vi "Write HDF5.vi"(4 "Append? [F]":bool, 6 "Igor Commands":string, 7 "path":path, 8 "error in (no error)":errorcluster, 9 "Comments":string, 10 "Data (Dictionary)":T1[](array[typedef]), 11 "LV to ITX.lvclass":refnum<class "LV to ITX.lvclass">) -> (0 "error out":errorcluster, 2 "path 2":path, 3 "LV to ITX.lvclass":refnum<class "LV to ITX.lvclass">)   [LabVIEW 2016, in "LV to ITX.lvclass"]
uses:
  LV to ITX.lvclass
  Typedefs/Dictionary--cluster.ctl
  <vilib>/addons/h5labview2/file/H5Fmode.ctl
  Typedefs/Filetype--enum.ctl
  LV to ITX.lvclass/LV to ITX.ctl
  <vilib>/addons/h5labview2/base/lib_path.vi
  <vilib>/addons/h5labview2/base/H5Equery.vi
  <vilib>/addons/h5labview2/base/hid_t.ctl
  <vilib>/addons/h5labview2/dataset/H5Dwrite.llb/H5Dwrite.xnode
  <vilib>/addons/h5labview2/file/H5F.lvlib
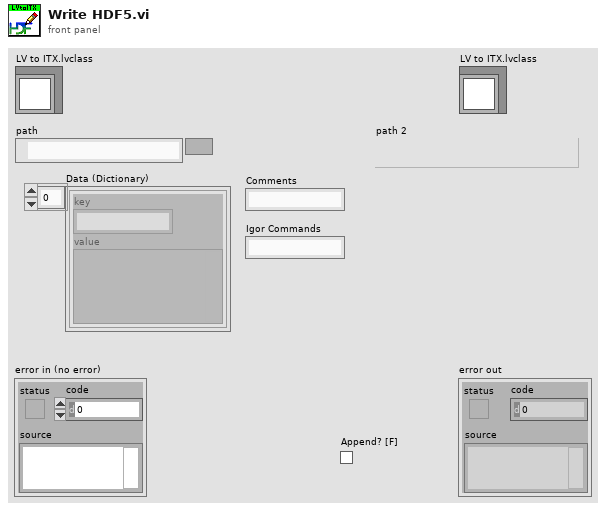
[diagram p1: front panel]
types:
  T1 = typedef "LV to ITX.lvclass/Dictionary--cluster.ctl" = cluster{"key":string, "value":variant}
  T2 = typedef "LV to ITX.lvclass/Filetype--enum.ctl" = enum16{"DAT", "ITX", "HDF5", "TDMS", "VI"}
  T3 = typedef "H5F.lvlib/H5Fmode.ctl" = enum16{"read-only", "read-write", "overwrite", "create new", "open or create"}
  T4 = typedef "hid_t.ctl" = i32
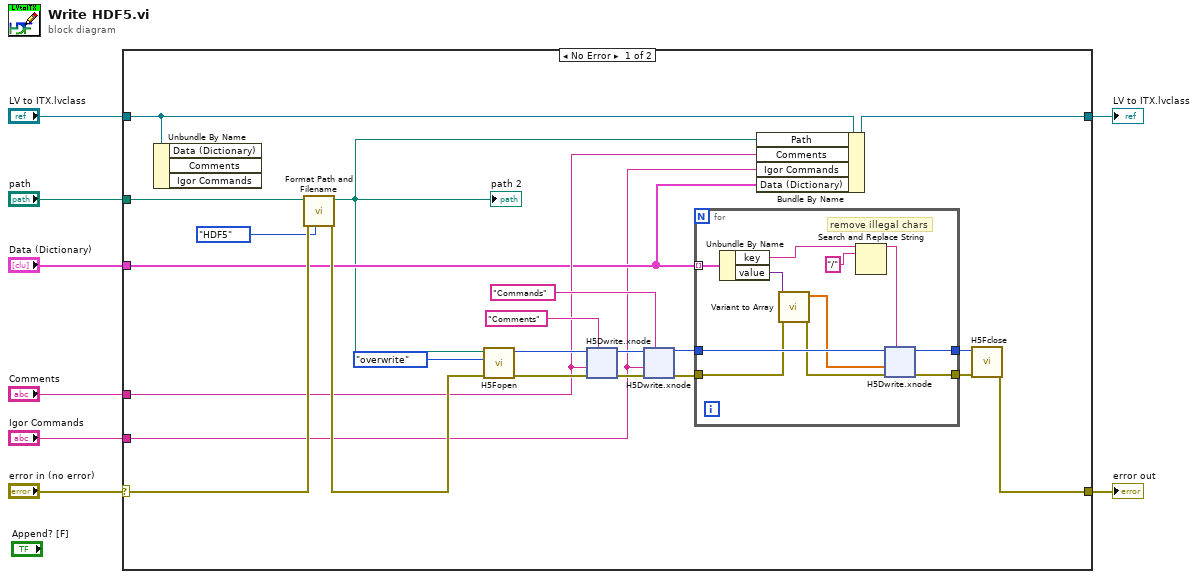
[diagram p0: block diagram]
diagram:
  n1 = case shown="No Error" "error in (no error)" {
    selector: "error in (no error)" -> [w18 w99]
    tunnel: [w23 w99] -> w6
    tunnel: "LV to ITX.lvclass" -> [w14 w100]
    tunnel: "path" -> [w16 _]
    tunnel: [w13 w100] -> w4
    tunnel: "Comments" -> [w12 _]
    tunnel: "Data (Dictionary)" -> [w11 _]
    tunnel: "Igor Commands" -> [w10 _]
    frame No Error {
      n2 = Unbundle By Name(w14) -> ()  [unwired: 3 out]
      n3 = call "Format Path and Filename.vi"("Type (TDMS)"=Filetype--enum."HDF5", "error in"=w18, "path"=w16) -> ("error out"=w17:errorcluster, "path"=w9:path)  [unwired: 6 in, 1 out]
      "path 2" <- w9
      n4 = call <vilib>:"H5Fopen.vi"("error in (no error)"=w17, "mode (read-only)"=H5Fmode."overwrite" ("mode"), "path"=w9) -> ("error out"=w19:errorcluster, "ref out"=w21:T4)  [unwired: 7 in]
      n5 = xnode "H5Dwrite.xnode"("dataset name"="Comments" ("attrib name"), "error in (no error)"=w19, "data"=w12, "ref in"=w21) -> ("error out"=w28:errorcluster, "ref out"=w27:T4)  [unwired: 3 in, 1 out]
      n6 = xnode "H5Dwrite.xnode"("dataset name"="Commands" ("attrib name"), "error in (no error)"=w28, "data"=w10, "ref in"=w27) -> ("error out"=w26:errorcluster, "ref out"=w24:T4)  [unwired: 3 in, 1 out]
      n7 = for {
        tunnel: w11 -> [w74] mode=indexing
        tunnel: w24 -> [w78]
        tunnel: [w77] -> w20
        tunnel: w26 -> [w70]
        tunnel: [w79] -> w22
        # "remove illegal chars"
        n8 = Unbundle By Name(w74) -> ("key"=w73:string, "value"=w72:variant)
        n9 = call "Variant to Array.vi"("error in (no error)"=w70, "value"=w72) -> ("error out"=w69:errorcluster, "1D Array"=w71:dbl[])  [unwired: 7 in, 1 out]
        n10 = Search and Replace String(input string=w73, search string="/") -> (result string=w76:string)  [unwired: 6 in, 3 out]
        n11 = xnode "H5Dwrite.xnode"("dataset name"=w76, "error in (no error)"=w69, "data"=w71, "ref in"=w78) -> ("error out"=w79:errorcluster, "ref out"=w77:T4)  [unwired: 3 in, 1 out]
      }
      n12 = Bundle By Name(cluster=w14, "Path"=w9, "Comments"=w12, "Igor Commands"=w10, "Data (Dictionary)"=w11) -> (w13:refnum<class "LV to ITX.lvclass">)
      n13 = call <vilib>:"H5Fclose.vi"("error in (no error)"=w22, "ref"=w20) -> ("error out"=w23:errorcluster)  [unwired: 9 in]
    }
    frame Error {
    }
  }
  "error out" <- w6
  "LV to ITX.lvclass" <- w4
